vi "Gyro.vi"() -> ()   [LabVIEW 2013]
doc: "Gyro Example\n\nThis VI shows the user how to open a channel to a Gyro, get an angle from a gyro, and reinitialize the gyro."
uses:
  <vilib>/Rock Robotics/SystemInterfaces/AI/FPGA_AIGyroChannel.ctl
  <vilib>/Rock Robotics/SystemInterfaces/Typedef/FPGA_TypedefAnalogModuleForGyro.ctl
panel:
  out "Voltage":dbl
  in  "Analog Module":T1
  in  "Gain (VoltsPerDegree/Second)":dbl=0.007
  in  "stop":bool
  out "Angle":dbl(knob) scale=0.0..360.0
  in  "Reset Zero Position":bool
  in  "Channel":T2
  # "This will display the current gyro angle."
  # "Wiring Diagram for Analog Breakout connected to an NI 9201"
  # "Set these inputs before running."
  # "This can be set while running."
  # "jumper to read battery or AI8"
  # "GND"
  # "SIG"
  # "5V"
  # "AI8\nAI7\nAI6\nAI5\nAI4\nAI3\nAI2\nAI1"
  # "Generic Gyro"
  # "+"
  # "12V from battery"
  # "-"
  # "\"power good\" LED"
  # "Specific Gyro Wiring:\nFor Analog Devices ADXRS401EB, ADXRS150EB and ADXRS300EB, wire RATEOUT to AI1 SIG (white PWM wire), wire AGND to AI1 GND (black PWM wire), and wire AVCC to AI1 5V (PWM red wire).  Also wire from AVCC to PDD.\n\nMost SparkFun Gyros wire according to the generic diagram"
  # "RATE"
  # "5V"
  # "GND"
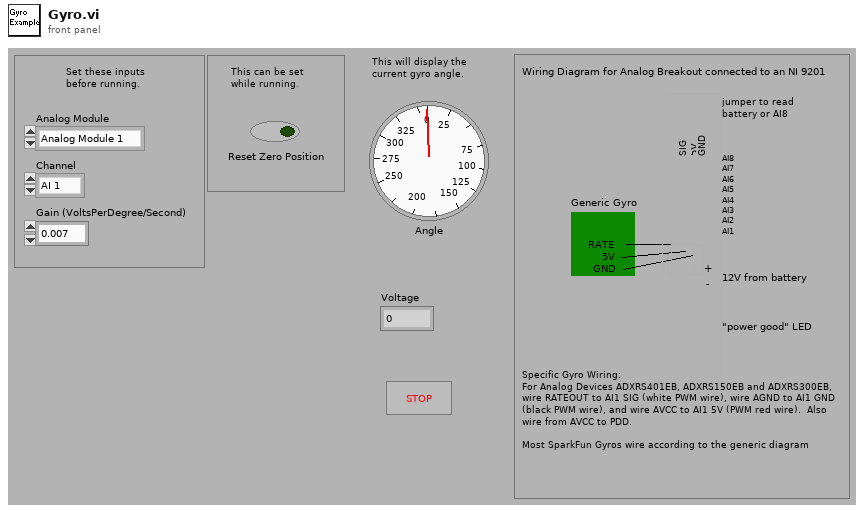
[diagram p1: front panel]
types:
  T1 = typedef "FPGA_TypedefAnalogModuleForGyro.ctl" = enum16{"Analog Module 1"}
  T2 = typedef "FPGA_AIGyroChannel.ctl" = enum8{"AI 1", "AI 2", "Invalid"}
  T3 = typedef "WPI_GyroDevRef.ctl" = cluster{"DevStatus":errorcluster, "Analog Module":T4, "Analog Channel":T5, "Offset":dbl, "Gain (VoltsPerDegree/Second)":dbl}
  T4 = typedef "FPGA_TypedefAnalogModule.ctl" = enum16{"Analog Module 1", "Analog Module 2"}
  T5 = typedef "FPGA_AIChannel.ctl" = enum8{"AI 1", "AI 2", "AI 3", "AI 4", "AI 5", "AI 6", "AI 7", "AI 8", "Invalid"}
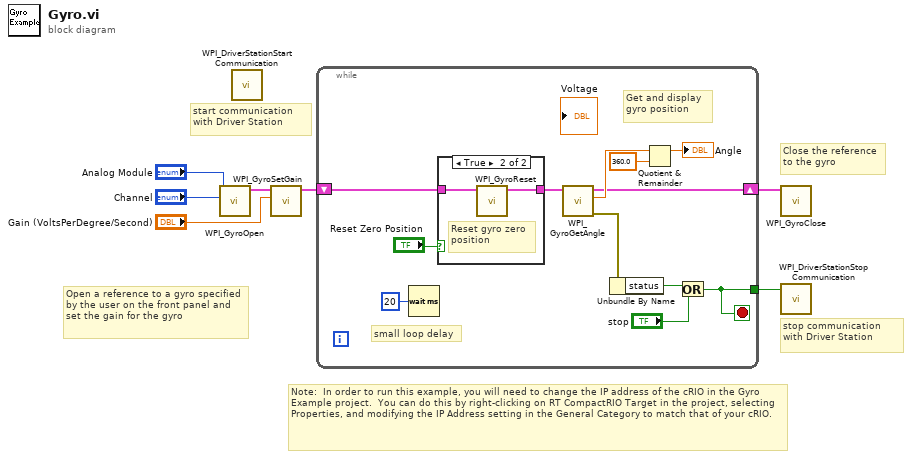
[diagram p0: block diagram]
diagram:
  # "stop communication with Driver Station"
  # "start communication with Driver Station"
  # "Note:  In order to run this example, you will need to change the IP address of the cRIO in the Gyro Example project.  You can do this by right-clicking on RT CompactRIO Target in the project, selecting Properties, and modifying the IP Address setting in the General Category to match that of your cRIO."
  # "Close the reference\nto the gyro"
  # "Open a reference to a gyro specified by the user on the front panel and set the gain for the gyro"
  n1 = call <vilib>:"WPI_GyroOpen.vi"("Analog Channel"="Channel", "Analog Module (Module 1)"="Analog Module") -> ("GyroDevRef"=w4:T3)  [unwired: 4 in, 5 out]
  n2 = call <vilib>:"WPI_DriverStationStart Communication.vi"() -> ()  [unwired: 1 in, 11 out]
  n3 = call <vilib>:"WPI_GyroSetGain.vi"("Gain (VoltsPerDegree/Second)"="Gain (VoltsPerDegree/Second)", "GyroDevRef"=w4) -> ("GyroDevRef"=w3:T3)  [unwired: 1 in, 8 out]
  n4 = while {
    shift-right: [w15] -> w6
    shift-left: w3 -> [w18]
    tunnel: [w13] -> w5
    stop <- w13 stop-if-true
    # "small loop delay"
    # "Get and display\ngyro position"
    n5 = Wait (ms)(milliseconds to wait=u32 20) -> ()  [unwired: 1 out]
    n6 = case shown="True" "Reset Zero Position" {
      tunnel: w18 -> [w20 w22]
      tunnel: [w20 w21] -> w17
      frame False {
      }
      frame True {
        # "Reset gyro zero \nposition"
        n7 = call <vilib>:"WPI_GyroReset.vi"("GyroDevRef"=w22) -> ("GyroDevRef"=w21:T3)  [unwired: 10 out]
      }
    }
    n8 = call <vilib>:"WPI_GyroGetAngle.vi"("GyroDevRef"=w17) -> ("error out"=w9:errorcluster, "Angle"=w16:dbl, "GyroDevRef"=w15:T3)  [unwired: 1 in, 7 out]
    n9 = Unbundle By Name(w9) -> ("status"=w14:bool)
    n10 = Quotient & Remainder(x=w16, y=360.0) -> (x-y*floor(x/y)=→"Angle":dbl)  [unwired: 1 out]
    n11 = Or(x=w14, y="stop") -> (x .or. y?=w13:bool)
  }
  n12 = call <vilib>:"WPI_GyroClose.vi"("GyroDevRef"=w6) -> ()  [unwired: 1 in, 10 out]
  n13 = call <vilib>:"WPI_DriverStationStop Communication.vi"("StopCommunication"=w5) -> ()  [unwired: 1 in, 10 out]
